vi "MC5e Open Config XML.vi"(8 "error in":errorcluster, 10 "default name":string="Get BLISS Config.XML") -> (0 "error out":errorcluster, 3 "value":string)   [LabVIEW 2020]
uses:
  MC5e Gobal_Variables.vi
  MC5e Global_Error_Codes.vi
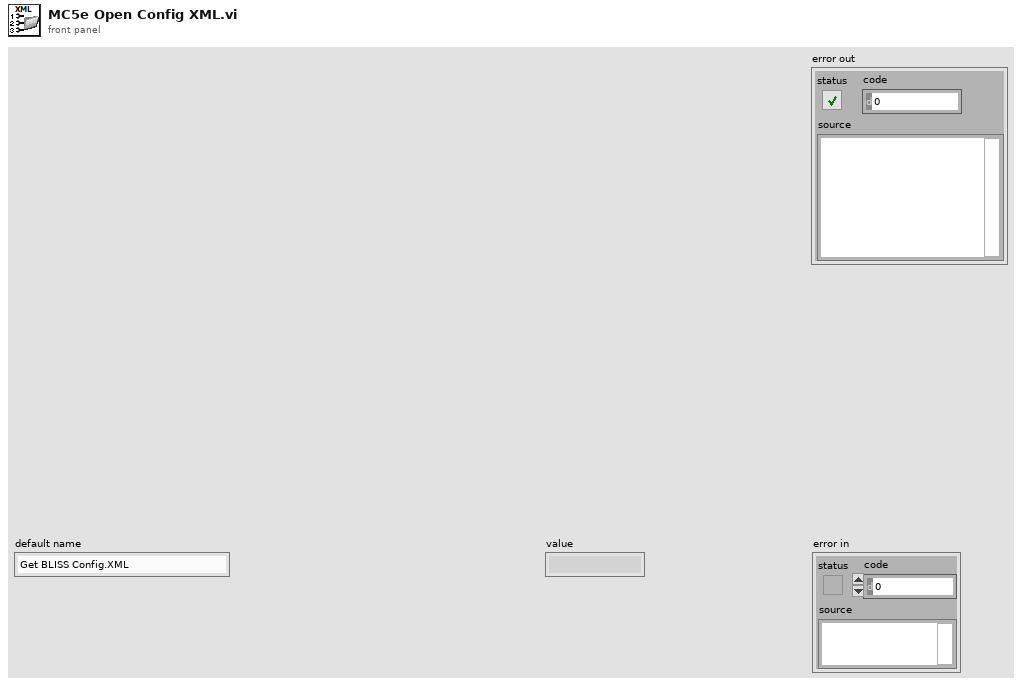
[diagram p1: front panel]
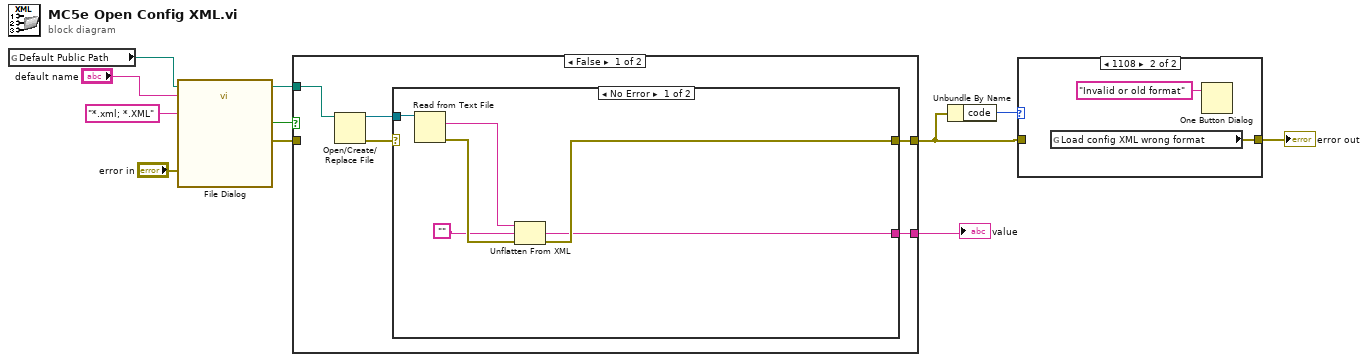
[diagram p0: block diagram]
diagram:
  n1 = global read "MC5e Gobal_Variables.vi" "Default Public Path"() -> (w3:path)
  n2 = call "File Dialog"("start path"=w3, "default name"="default name", "error in"="error in", "pattern (all files)"="*.xml; *.XML") -> ("selected path"=w8:path, "cancelled"=w10:bool, "error out"=w7:errorcluster)  [unwired: 8 in, 1 out]
  n3 = case shown="False" w10 {
    tunnel: [w16 w24] -> w4
    tunnel: w8 -> [w15 _]
    tunnel: w7 -> [_ w24]
    tunnel: [w12 _] -> w1
    frame False {
      n4 = Open/Create/Replace File(file path (use dialog)=w15) -> (refnum out=w13:refnum<file>, error out=w14:errorcluster)  [unwired: 5 in, 1 out]
      n5 = case shown="No Error" w14 {
        selector: w14 -> [_ w23]
        tunnel: [w22 w23] -> w16
        tunnel: w13 -> [w21 _]
        tunnel: [w17 _] -> w12
        frame No Error {
          n6 = Read from Text File(file (use dialog)=w21) -> (text=w20:string, error out=w19:errorcluster)  [unwired: 3 in, 2 out]
          n7 = Unflatten From XML(xml string=w20, type="", error in (no error)=w19) -> (value=w17:string, error out=w22:errorcluster)
        }
        frame Error {
        }
      }
    }
    frame True {
    }
  }
  "value" <- w1
  n8 = Unbundle By Name(w4) -> ("code"=w6:i32)
  n9 = case shown="1108" w6 {
    tunnel: [w25 w27] -> w5
    tunnel: w4 -> [w25 _]
    frame 0, Default {
    }
    frame 1108 {
      n10 = global read "MC5e Global_Error_Codes.vi" "Load config XML wrong format"() -> (w27:errorcluster)
      n11 = One Button Dialog(message="Invalid or old format") -> ()  [unwired: 1 in, 1 out]
    }
  }
  "error out" <- w5
